vi "Basic Operations (string).vi"(8 "Operation":T1, 10 "x":string, 11 "y":string) -> (3 "x op y":string)   [LabVIEW 2024, in "Libreria de reuso.lvlib"]
uses:
  Libreria de reuso.lvlib
  Operation--enum.ctl
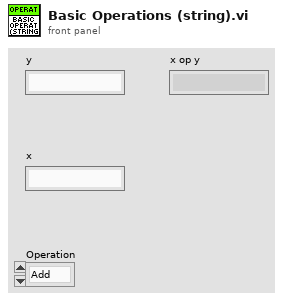
[diagram p1: front panel]
types:
  T1 = typedef "Libreria de reuso.lvlib/Operation--enum.ctl" = enum16{"Add", "Subtract", "Multiply", "Divide"}
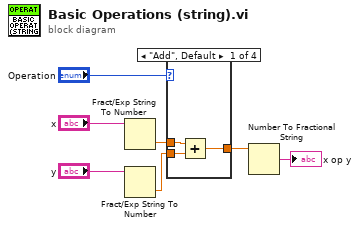
[diagram p0: block diagram]
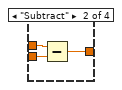
[diagram p2: hidden frame]
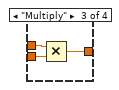
[diagram p3: hidden frame]
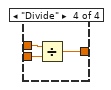
[diagram p4: hidden frame]
diagram:
  n1 = Fract/Exp String To Number(string="x") -> (number=w3:dbl)  [unwired: 3 in, 1 out]
  n2 = Fract/Exp String To Number(string="y") -> (number=w2:dbl)  [unwired: 3 in, 1 out]
  n3 = case shown="\"Add\", Default" "Operation" {
    tunnel: w2 -> [w10 w13 w16 w19]
    tunnel: w3 -> [w9 w12 w15 w18]
    tunnel: [w8 w11 w14 w17] -> w5
    frame "Add", Default {
      n4 = Add(x=w9, y=w10) -> (x+y=w8:dbl)
    }
    frame "Subtract" {
      n5 = Subtract(x=w12, y=w13) -> (x-y=w11:dbl)
    }
    frame "Multiply" {
      n6 = Multiply(x=w15, y=w16) -> (x*y=w14:dbl)
    }
    frame "Divide" {
      n7 = Divide(x=w18, y=w19) -> (x/y=w17:dbl)
    }
  }
  n8 = Number To Fractional String(number=w5) -> (F-format string=→"x op y":string)  [unwired: 3 in]
